vi "Timed_loop_SDI-12_automation.vi"(10 "VISA resource name to start measurement":refnum<visa-resource-name>="ASRL4::INSTR", 11 "VISA resource name to write the measurement on to a file":refnum<visa-resource-name>="ASRL4::INSTR") -> (2 "second indicator":bool=TRUE, 3 "FIle is succesfully saved":bool=TRUE)   [LabVIEW 2019]
uses:
  <vilib>/platform/TimedLoop/XDataNode/XDataNode.xnode
  <vilib>/Platform/TimedLoop/XDataNode/nitl_modes.ctl
  <vilib>/Platform/TimedLoop/XDataNode/XDNodeRunTimeDep.lvlib
  <vilib>/Platform/TimedLoop/XDataNode/wakeup.ctl
  <vilib>/Platform/TimedLoop/XDataNode/timing_clust.ctl
  <vilib>/Instr/_visa.llb/VISA Configure Serial Port (Instr).vi
  LabVIEW Data/Hemanth_myRIO/Control 1.ctl
  <vilib>/myRIO/Express VI/Onboard Devices/LED/LED Express VI.xnode
  <vilib>/myRIO/Common/Instrument Driver Framework/myRIO v1.0/DIO/typedefs/DIO Channels Enum.ctl
  <vilib>/myRIO/Common/Instrument Driver Framework/myRIO v1.0/DIO/typedefs/DIO Channels List.ctl
  <vilib>/myRIO/Common/Instrument Driver Framework/Utilities/typedefs/Generic FPGA Reference.ctl
  <vilib>/myRIO/Common/Instrument Driver Framework/Utilities/typedefs/myRIO v1.0 Reference.ctl
  <vilib>/myRIO/Common/Instrument Driver Framework/Utilities/typedefs/Hardware Version Enum.ctl
  <vilib>/myRIO/Common/Instrument Driver Framework/Utilities/typedefs/myRIO Generic Hardware Reference.ctl
  <vilib>/myRIO/Instrument Drivers/Onboard IO/DIO/vis/myRIO DIO Open.xnode
  <vilib>/myRIO/Common/Instrument Driver Framework/Utilities/vis/Is FPGA Ref Available.vi
  <vilib>/myRIO/Common/Instrument Driver Framework/myRIO v1.0/DIO/vis/myRIO v1.1 Open DIO.vi
  <vilib>/userdefined/High Color/nirio_resource_hc.ctl
  <vilib>/myRIO/Instrument Drivers/Onboard IO/DIO/typedefs/DIO Reference.ctl
  <vilib>/myRIO/Instrument Drivers/Onboard IO/DIO/DIO.lvlib
  <vilib>/myRIO/Instrument Drivers/Onboard IO/DIO/vis/Write.vi
panel:
  out "Response 2":string
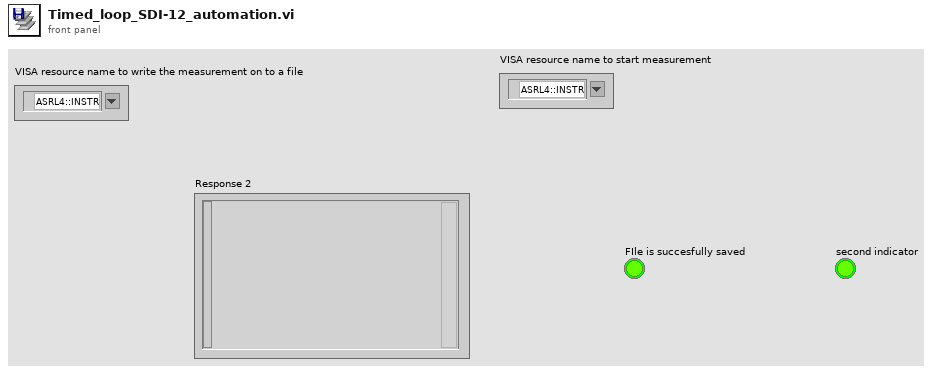
[diagram p1: front panel]
types:
  T1 = enum16{"open", "replace", "create", "open or create", "replace or create", "replace or create with confirmation"}
  T2 = typedef "XDNodeRunTimeDep.lvlib/timing_clust.ctl" = cluster{"Expected End [f-1]":u64, "Actual End [f-1]":u64, "Finished Late? [f-1]":bool, "Expected End [i-1]":u64, "Actual End [i-1]":u64, "Finished Late? [i-1]":bool, "Expected Start [i]":u64, "Actual Start [i]":u64, "Expected Start [f]":u64, "Actual Start [f]":u64, "Source Name":string, "Structure Name":string, "Period":i64, "Deadline":i64, "Offset":i64, "Start":i64, "Priority":i32, "Timeout":i32, "Mode":T3, "Wakeup Reason":T4, "Error":errorcluster, "Source Type":string, "Secondary Source Type":string, "Global End Time":u64, "Global Start Time":u64, "Frame Duration":u64, "Iteration Duration":u64, "Assigned CPU":i32, "I/O Scan Engine Mode":u32}
  T3 = typedef "XDNodeRunTimeDep.lvlib/nitl_modes.ctl" = enum32{"No Change", "Process missed periods, maintain original phase", "Discard missed periods, maintain original phase", "Process missed periods, ignore original phase", "Discard missed periods, ignore original phase"}
  T4 = typedef "XDNodeRunTimeDep.lvlib/wakeup.ctl" = enum32{"Normal", "Aborted", "Asynchronous wakeup", "Timing source error", "Timed loop error", "Timeout"}
  T5 = typedef "Control 1.ctl" = enum16{"NUL", "SOH", "STX", "ETX", "EOT", "ENQ", "ACK", "BEL", "BS", "HT", "LF", "VT", "FF", "CR", "SO", "SI", "DLE", "DC1", "DC2", "DC3", "DC4", "NAK", "SYN", "ETB", "CAN", "EM", "SUB", "ESC", "FS", "GS", "RS", "US", "SP", "!", "\"", "#", "$", "%", "&", "'", "(", ")", "*", "+", ",", "- (-)", ".", "/", "0", "1", "2", "3", "4", "5", "6", "7", "8", "9", ":", ";", "<", "=", ">", "?", "@", "A", "B", "C", "D", "E", "F", "G", "H", "I", "J", "K", "L", "M", "N", "O", "P", "Q", "R", "S", "T", "U", "V", "W", "X", "Y", "Z", "[", "\\", "]", "^", "_", "`", "a", "b", "c", "d", "e", "f", "g", "h", "i", "j", "k", "l", "m", "n", "o", "p", "q", "r", "s", "t", "u", "v", "w", "x", "y", "z", "{", "|", "}", "~"}
  T6 = typedef "DIO.lvlib/DIO Reference.ctl" = cluster{"myRIO Reference":T7, "DIO Channels List":T11}
  T7 = typedef "myRIO Generic Hardware Reference.ctl" = cluster{"myRIO Model":T8, "myRIO Hardware Reference":T9}
  T8 = typedef "Hardware Version Enum.ctl" = enum16{"Unknown", "myRIO-1900", "myRIO-1950", "roboRIO", "NI ELVIS RIO CM", "ELVIS III"}
  T9 = typedef "myRIO v1.0 Reference.ctl" = cluster{"Generic FPGA Reference":T10, "Allow multiple opens":bool}
  T10 = typedef "Generic FPGA Reference.ctl" = refnum<k20>
  T11 = typedef "DIO Channels List.ctl" = T12[]
  T12 = typedef "DIO Channels Enum.ctl" = enum16{"Not Connected", "C/DIO0", "C/DIO1", "C/DIO2", "C/DIO3", "C/DIO4", "C/DIO5", "C/DIO6", "C/DIO7", "A/DIO0", "A/DIO1", "A/DIO2", "A/DIO3", "A/DIO4", "A/DIO5", "A/DIO6", "A/DIO7", "A/DIO8", "A/DIO9", "A/DIO10", "A/DIO11", "A/DIO12", "A/DIO13", "A/DIO14", "A/DIO15", "A/DIO16", "A/DIO17", "A/DIO18", "A/DIO19", "B/DIO0", "B/DIO1", "B/DIO2", "B/DIO3", "B/DIO4", "B/DIO5", "B/DIO6", "B/DIO7", "B/DIO8", "B/DIO9", "B/DIO10", "B/DIO11", "B/DIO12", "B/DIO13", "B/DIO14", "B/DIO15", "B/DIO16", "B/DIO17", "B/DIO18", "B/DIO19", "LED0", "LED1", "LED2", "LED3", "Button0", "DIO/DIO0", "DIO/DIO1", "DIO/DIO2", "DIO/DIO3", "DIO/DIO4", "DIO/DIO5", "DIO/DIO6", "DIO/DIO7", "DIO/DIO8", "DIO/DIO9", "SPI/CS0", "SPI/CS1", "SPI/CS2", "SPI/CS3", "LED RADIO (Green)", "LED RADIO (Red)", "LED COMM (Green)", "LED COMM (Red)", "LED MODE (Green)", "LED MODE (Red)"}
  T13 = typedef "nirio_resource_hc.ctl" = tag
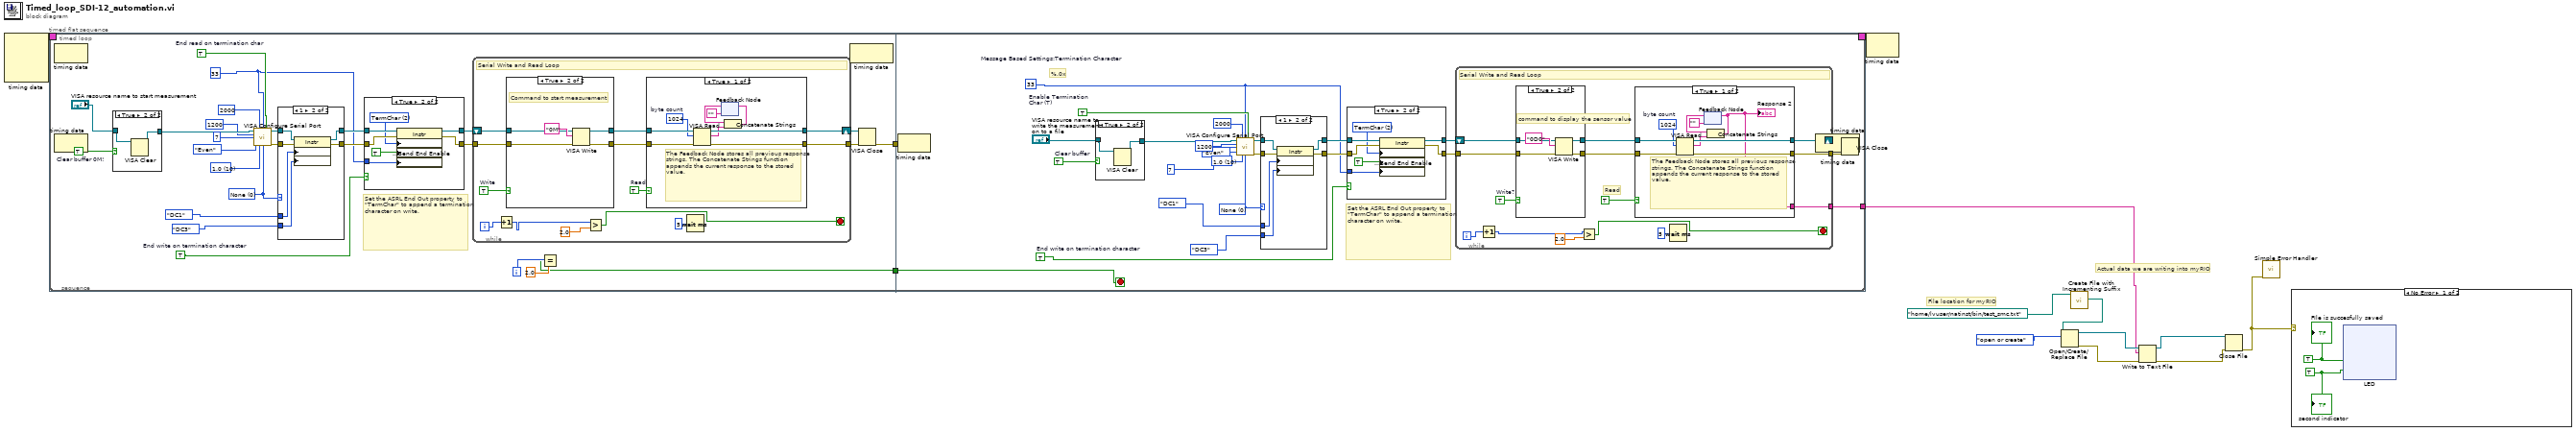
[diagram p0: block diagram]
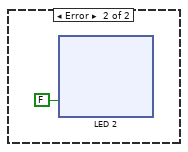
[diagram p2: hidden frame]
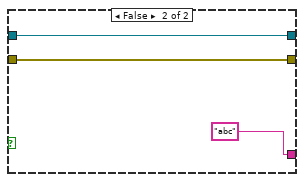
[diagram p12: hidden frame]
diagram:
  # "Actual data we are writing into myRIO"
  # "File location for myRIO"
  n1 = node-c288() -> (w11:T2)  [unwired: 4 in]
  n2 = timed-loop {
    timing: w11 -> [_]
    timing-out: [_] -> w10
    tunnel: [w12] -> w4
    i -> [w28]
    stop <- w107 stop-if-true
    n3 = timed-sequence {
      timing: _ -> [_]
      timing-out: _ -> [_]
      tunnel: [w13] -> w12
      n4 = timed-flat-sequence {
        tunnel: [w30] -> w15
        tunnel: [w27] -> w14
        tunnel: w15 -> [_]
        tunnel: w14 -> [w107]
        tunnel: [w106] -> w13
        frame #0 {
          w18 = u8 33 ("Message Based Settings:Termination Character")
          w19 = u16 0 items=["None", "XON/XOFF", "RTS/CTS", "XON/XOFF & RTS/CTS", "DTR/DSR", "XON/XOFF & DTR/DSR"] ("flow control (0:none)")
          w20 = u16 10 items=["1.0"=10, "1.5"=15, "2.0"=20] ("stop bits (10: 1 bit)")
          w24 = TRUE  # Clear buffer 0M!
          w25 = TRUE  # End write on termination character
          w26 = TRUE  # End read on termination char
          # "Set the ASRL End Out property to \"TermChar\" to append a termination character on write."
          n5 = node-c288() -> ()  [unwired: 1 in, 1 out]
          n6 = case shown="True" w24 {
            tunnel: "VISA resource name to start measurement" -> [w42 w44]
            tunnel: [w42 w43] -> w32
            frame False {
            }
            frame True {
              n7 = VISA Clear(VISA resource name=w44) -> (VISA resource name out=w43:refnum<visa-resource-name>)  [unwired: 1 in, 1 out]
            }
          }
          n8 = call-poly "VISA Configure Serial Port"("VISA resource name"=w32, "timeout (10sec)"=u32 2000, "termination char\n(0xA = '\\n' = LF)"=w18, "Enable Termination\nChar (T)"=w26, "baud rate (9600)"=u32 1200, "data bits (8)"=u16 7, "parity (0:none)"=enum16{"None", "Odd", "Even", "Mark", "Space"}."Even", "stop bits (10: 1 bit)"=w20, "flow control (0:none)"=w19) -> ("VISA resource name out"=w40:refnum<visa-resource-name>, "error out"=w41:errorcluster)  [unwired: 1 in, 4 out]
          n9 = case shown="1" w19 {
            tunnel: [w54 w61] -> w37
            tunnel: [w55 w60] -> w35
            tunnel: w41 -> [w54 w59]
            tunnel: w40 -> [w55 w58]
            tunnel: Control_1."DC1" ("XON") -> [_ w57]
            tunnel: Control_1."DC3" ("XOFF") -> [_ w56]
            frame Default {
            }
            frame 1 {
              n10 = property class="Instr"(reference=w58, error in=w59, "Serial Settings:Flow Control XON Character"=w57, "Serial Settings:Flow Control XOFF Character"=w56) -> (reference out=w60:refnum<visa-resource-name>, error out=w61:errorcluster)
            }
          }
          n11 = case shown="True" w25 {
            tunnel: w35 -> [w45 w53]
            tunnel: w37 -> [w46 w52]
            tunnel: [w45 w51] -> w34
            tunnel: [w46 w50] -> w36
            tunnel: w18 -> [_ w47]
            frame False {
            }
            frame True {
              w49 = u16 2 items=["None", "LastBit", "TermChar", "Break"] ("Serial Settings:Serial End Mode for Writes")
              n12 = property class="Instr"(reference=w53, error in=w52, "Serial Settings:End Mode for Writes"=w49, "Message Based Settings:Send End Enable"=TRUE, "Message Based Settings:Termination Character"=w47) -> (reference out=w51:refnum<visa-resource-name>, error out=w50:errorcluster)
            }
          }
          n13 = while {
            shift-right: [w74] -> w38
            shift-left: w34 -> [w73]
            tunnel: w36 -> [w72]
            tunnel: [w68] -> w39
            i -> [w67]
            stop <- w64 stop-if-true
            w62 = TRUE  # Read
            w63 = TRUE  # Write
            # "Serial Write and Read Loop"
            n14 = Increment(x=w67) -> (x+1=w65:i32)
            n15 = case shown="True" w63 {
              tunnel: w73 -> [w76 w80]
              tunnel: w72 -> [w75 w79]
              tunnel: [w76 w78] -> w71
              tunnel: [w75 w77] -> w70
              frame False {
              }
              frame True {
                # "Command to start measurement"
                n16 = VISA Write(VISA resource name=w80, write buffer="0M" ("Command"), error in (no error)=w79) -> (VISA resource name out=w78:refnum<visa-resource-name>, error out=w77:errorcluster)  [unwired: 1 out]
              }
            }
            n17 = Greater?(x=w65, y=2.0) -> (0:w64:bool)
            n18 = case shown="True" w62 {
              tunnel: [w88 w92] -> w74
              tunnel: w71 -> [w90 w92]
              tunnel: [w87 w91] -> w68
              tunnel: w70 -> [w89 w91]
              frame True {
                w82 = u32 1024  # byte count
                # "The Feedback Node stores all previous response strings. The Concatenate Strings function appends the current response to the stored value."
                n19 = VISA Read(VISA resource name=w90, byte count=w82, error in (no error)=w89) -> (VISA resource name out=w88:refnum<visa-resource-name>, read buffer=w86:string, error out=w87:errorcluster)  [unwired: 1 out]
                n20 = feedback #1("") -> (w85:string)
                n21 = Concatenate Strings(w85, w86) -> (w84:string)
                n22 = feedback-in #1(w84) -> ()
              }
              frame False {
              }
            }
            n23 = Wait (ms)(milliseconds to wait=u32 5) -> ()  [unwired: 1 out]
          }
          n24 = Equal?(x=w28, y=2.0) -> (x = y?=w27:bool)
          n25 = node-c288() -> ()  [unwired: 1 in, 1 out]
          n26 = VISA Close(VISA resource name=w38, error in (no error)=w39) -> (error out=w30:errorcluster)
        }
        frame #1 {
          w97 = u16 0 items=["None", "XON/XOFF", "RTS/CTS", "XON/XOFF & RTS/CTS", "DTR/DSR", "XON/XOFF & DTR/DSR"] ("flow control (0:none)")
          w98 = u16 10 items=["1.0"=10, "1.5"=15, "2.0"=20] ("stop bits (10: 1 bit)")
          w102 = u8 33  # Message Based Settings:Termination Character
          w103 = TRUE  # End write on termination character
          w104 = TRUE  # Enable Termination Char (T)
          w105 = TRUE  # Clear buffer
          # "%.0x"
          # "Set the ASRL End Out property to \"TermChar\" to append a termination character on write."
          n27 = node-c288() -> ()  [unwired: 1 in, 1 out]
          n28 = case shown="True" w105 {
            tunnel: "VISA resource name to write the measurement on to a file" -> [w119 w121]
            tunnel: [w119 w120] -> w109
            frame False {
            }
            frame True {
              n29 = VISA Clear(VISA resource name=w121) -> (VISA resource name out=w120:refnum<visa-resource-name>)  [unwired: 1 in, 1 out]
            }
          }
          n30 = call-poly "VISA Configure Serial Port"("VISA resource name"=w109, "timeout (10sec)"=u32 2000, "termination char\n(0xA = '\\n' = LF)"=w102, "Enable Termination\nChar (T)"=w104, "baud rate (9600)"=u32 1200, "data bits (8)"=u16 7, "parity (0:none)"=enum16{"None", "Odd", "Even", "Mark", "Space"}."Even", "stop bits (10: 1 bit)"=w98, "flow control (0:none)"=w97) -> ("VISA resource name out"=w117:refnum<visa-resource-name>, "error out"=w118:errorcluster)  [unwired: 1 in, 4 out]
          n31 = case shown="1" w97 {
            tunnel: [w131 w138] -> w114
            tunnel: [w132 w137] -> w112
            tunnel: w118 -> [w131 w136]
            tunnel: w117 -> [w132 w135]
            tunnel: Control_1."DC1" ("XON") -> [_ w134]
            tunnel: Control_1."DC3" ("XOFF") -> [_ w133]
            frame Default {
            }
            frame 1 {
              n32 = property class="Instr"(reference=w135, error in=w136, "Serial Settings:Flow Control XON Character"=w134, "Serial Settings:Flow Control XOFF Character"=w133) -> (reference out=w137:refnum<visa-resource-name>, error out=w138:errorcluster)
            }
          }
          n33 = case shown="True" w103 {
            tunnel: w112 -> [w122 w130]
            tunnel: w114 -> [w123 w129]
            tunnel: [w122 w128] -> w111
            tunnel: [w123 w127] -> w113
            tunnel: w102 -> [_ w125]
            frame False {
            }
            frame True {
              w126 = u16 2 items=["None", "LastBit", "TermChar", "Break"] ("Serial Settings:Serial End Mode for Writes")
              n34 = property class="Instr"(reference=w130, error in=w129, "Serial Settings:End Mode for Writes"=w126, "Message Based Settings:Send End Enable"=TRUE, "Message Based Settings:Termination Character"=w125) -> (reference out=w128:refnum<visa-resource-name>, error out=w127:errorcluster)
            }
          }
          n35 = while {
            shift-right: [w152] -> w115
            shift-left: w111 -> [w151]
            tunnel: w113 -> [w150]
            tunnel: [w146] -> w116
            tunnel: [w141] -> w106
            i -> [w145]
            stop <- w142 stop-if-true
            w140 = TRUE  # Write?
            # "Read"
            # "Serial Write and Read Loop"
            n36 = Increment(x=w145) -> (x+1=w143:i32)
            n37 = case shown="True" w140 {
              tunnel: w151 -> [w154 w158]
              tunnel: w150 -> [w153 w157]
              tunnel: [w154 w156] -> w149
              tunnel: [w153 w155] -> w148
              frame False {
              }
              frame True {
                # "command to display the sensor value"
                n38 = VISA Write(VISA resource name=w158, write buffer="0D0" ("Command 2"), error in (no error)=w157) -> (VISA resource name out=w156:refnum<visa-resource-name>, error out=w155:errorcluster)  [unwired: 1 out]
              }
            }
            n39 = Greater?(x=w143, y=2.0) -> (0:w142:bool)
            n40 = case shown="True" TRUE {
              tunnel: [w166 w171] -> w152
              tunnel: w149 -> [w168 w171]
              tunnel: [w165 w170] -> w146
              tunnel: w148 -> [w167 w170]
              tunnel: [w161 "abc"] -> w141
              frame True {
                w160 = u32 1024  # byte count
                # "The Feedback Node stores all previous response strings. The Concatenate Strings function appends the current response to the stored value."
                n41 = VISA Read(VISA resource name=w168, byte count=w160, error in (no error)=w167) -> (VISA resource name out=w166:refnum<visa-resource-name>, read buffer=w164:string, error out=w165:errorcluster)  [unwired: 1 out]
                n42 = feedback #2("") -> (w163:string)
                n43 = Concatenate Strings(w163, w164) -> (w161:string)
                "Response 2" <- w161
                n44 = feedback-in #2(w161) -> ()
              }
              frame False {
              }
            }
            n45 = Wait (ms)(milliseconds to wait=u32 5) -> ()  [unwired: 1 out]
          }
          n46 = node-c288() -> ()  [unwired: 1 in, 1 out]
          n47 = VISA Close(VISA resource name=w115, error in (no error)=w116) -> ()  [unwired: 1 out]
        }
      }
    }
    n48 = node-c288() -> ()  [unwired: 1 in, 1 out]
    n49 = node-c288() -> ()  [unwired: 1 in, 1 out]
  }
  n50 = node-c288(w10) -> ()  [unwired: 1 out]
  n51 = call <vilib>:"Create File with Incrementing Suffix.vi"("file path"=path "/home/lvuser/natinst/bin/test_smc.txt" ("file path (use dialog)")) -> ("actual path"=w2:path)  [unwired: 8 in, 2 out]
  n52 = Open/Create/Replace File(file path (use dialog)=w2, operation (0:open)=T1."open or create") -> (refnum out=w8:refnum<file>, error out=w7:errorcluster)  [unwired: 4 in, 1 out]
  n53 = Write to Text File(file (use dialog)=w8, text=w4, error in=w7) -> (refnum out=w6:refnum<file>, error out=w5:errorcluster)  [unwired: 1 in, 1 out]
  n54 = Close File(refnum=w6, error in=w5) -> (error out=w1:errorcluster)  [unwired: 1 out]
  n55 = call <vilib>:"Simple Error Handler.vi"("error in (no error)"=w1) -> ()  [unwired: 4 in, 5 out]
  n56 = case shown="No Error" w1 {
    frame No Error {
      w176 = TRUE ("LED1")
      w177 = TRUE ("LED0")
      n57 = xnode "LED"("LED0"=w177, "LED1"=w176) -> ()  [unwired: 1 in, 1 out]
      "FIle is succesfully saved" <- w177
      "second indicator" <- w176
    }
    frame Error {
      n58 = xnode "LED 2"("LED0"=FALSE) -> ()  [unwired: 1 in, 1 out]
    }
  }
